vi "Coersion dot.vi"() -> ()   [LabVIEW 2020]
panel:
  in  "Numeric 6":i8
  out "Numeric 5":u8
  out "Numeric 4":u8
  in  "Numeric 2":i8
  # "Coersion dot"
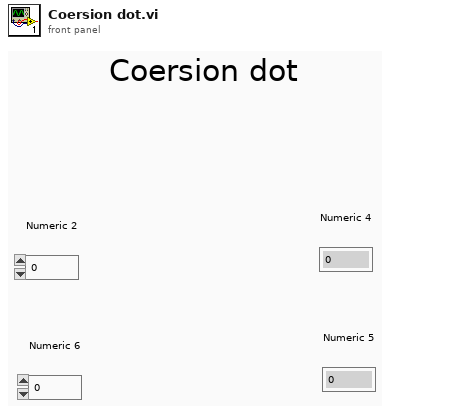
[diagram p1: front panel]
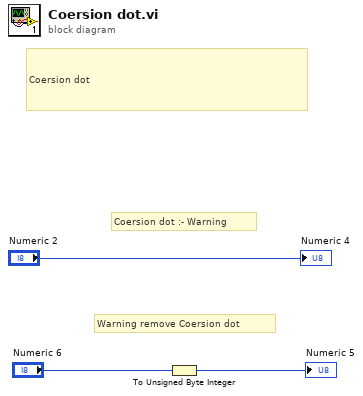
[diagram p0: block diagram]
diagram:
  # "Coersion dot"
  # "Warning remove Coersion dot"
  # "Coersion dot :- Warning"
  n1 = To Unsigned Byte Integer(number="Numeric 6") -> (unsigned 8bit integer=→"Numeric 5":u8)
  "Numeric 4" <- "Numeric 2"
